vi "Approach States Angle.vi"() -> ()   [LabVIEW 2017]
panel:
  out "Next Forearm Angle":dbl format="%#_13g"
  out "Next Backarm Angle":dbl format="%#_13g"
  in  "Current Forearm Angle":dbl
  in  "Moving Forward?":bool=TRUE
  in  "Current Backarm Angle":dbl
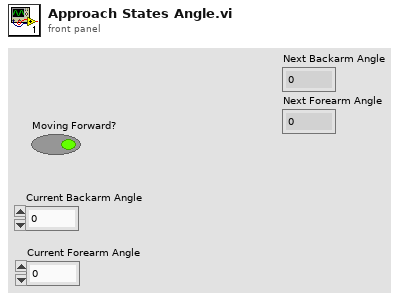
[diagram p1: front panel]
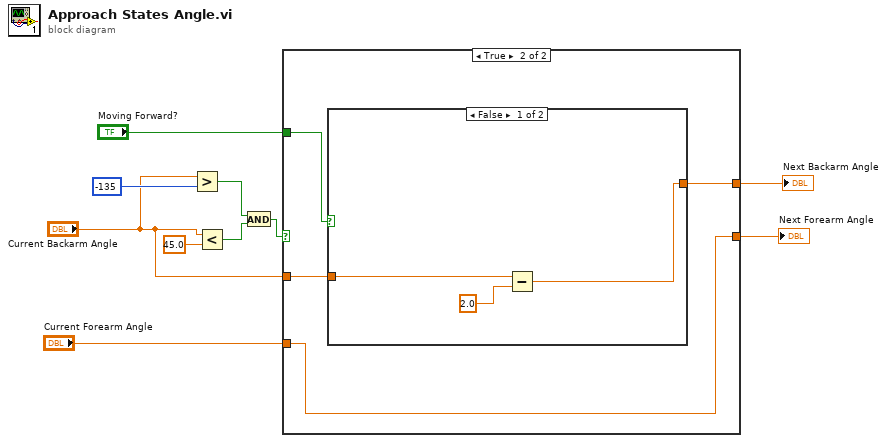
[diagram p0: block diagram]
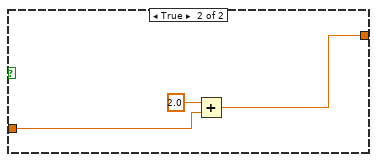
[diagram p4: hidden frame]
diagram:
  n1 = Greater?(x="Current Backarm Angle", y=-135) -> (0:w5:bool)
  n2 = Less?(x="Current Backarm Angle", y=45.0) -> (x < y?=w4:bool)
  n3 = And(x=w5, y=w4) -> (x .and. y?=w6:bool)
  n4 = case shown="True" w6 {
    tunnel: "Current Forearm Angle" -> [_ w14]
    tunnel: [_ w14] -> w8
    tunnel: "Moving Forward?" -> [_ w13]
    tunnel: "Current Backarm Angle" -> [_ w12]
    tunnel: [_ w11] -> w1
    frame False {
      n5 = case shown="True" {
        selector: _ -> [_ _]
        frame False {
        }
        frame True {
        }
      }
    }
    frame True {
      n6 = case shown="False" w13 {
        tunnel: w12 -> [w17 w19]
        tunnel: [w15 w18] -> w11
        frame False {
          n7 = Subtract(x=w17, y=2.0) -> (x-y=w15:dbl)
        }
        frame True {
          n8 = Add(x=2.0, y=w19) -> (x+y=w18:dbl)
        }
      }
    }
  }
  "Next Backarm Angle" <- w1
  "Next Forearm Angle" <- w8
